vi "demodrive.vi"   [LabVIEW 2012, in "Demo.lvrbt"]
uses:
  Demo.lvrbt
  <vilib>/NXT/Hardware/Plugins/Tetrix DC Motor/TetrixDCMotorAddress.ctl
  <vilib>/FTC/FTC Read Controller Packet.vi
  <vilib>/FTC/FTC Read Button States.vi
  <vilib>/FTC/FTC Calculate Drive Power - Tank.vi
  <vilib>/NXT/NXTIO Xnodes/NXTIONodeSubVIs/TETRIX IO Move DC Motors.vi
  <vilib>/NXT/NXTIO Xnodes/NXTIONodeSubVIs/TETRIX IO Check Battery.vi
  <vilib>/NXT/NXTIO Xnodes/AddressXNode/NXTIOAddress.xnode
  <vilib>/NXT/Subs/LVHSConnector.ctl
  <vilib>/NXT/NXTIO Xnodes/NXTIOXNode/NXTIO.xnode
  <vilib>/NXT/LegoClasses/BrickReference/BrickReference.lvclass
panel:
  # "This VI was generated based on your configuration in the Remote Control Editor. You may modify the code as needed for your robot. To test this program for an FTC match, return to the Remote Control Editor, select the \"Run Program\" tab, and choose \"FTC Game\"."
types:
  T1 = typedef "TetrixDCMotorAddress.ctl" = i16
  T2 = cluster{"TetrixDCMotor":T1, "TetrixDCMotor 2":T1}
  T3 = typedef "LVHSConnector.ctl" = refnum<class "BrickReference.lvclass">
  T4 = typedef "FTC ControllerState.ctl" = cluster{"Left X":i8, "Left Y":i8, "Right X":i8, "Right Y":i8, "Button Encoding 9-12":u8, "Button Encoding 1-8":u8, "POV":T5}
  T5 = typedef "FTC POVState.ctl" = i8
  T6 = typedef "FTC ButtonEventType.ctl" = enum16{"Pressed", "Released"}
  T7 = cluster{"Button ID":enum16{"None", "Button 1", "Button 2", "Button 3", "Button 4", "Button 5", "Button 6", "Button 7", "Button 8", "Button 9", "Button 10", "Button 11", "Button 12", "POV Up", "POV Up Right", "POV Right", "POV Down Right", "POV Down", "POV Down Left", "POV Left", "POV Up Left"}, "Event Type":T6}[]
  T8 = enum16{"None", "Button 1", "Button 2", "Button 3", "Button 4", "Button 5", "Button 6", "Button 7", "Button 8", "Button 9", "Button 10", "Button 11", "Button 12", "POV Up", "POV Up Right", "POV Right", "POV Down Right", "POV Down", "POV Down Left", "POV Left", "POV Up Left"}
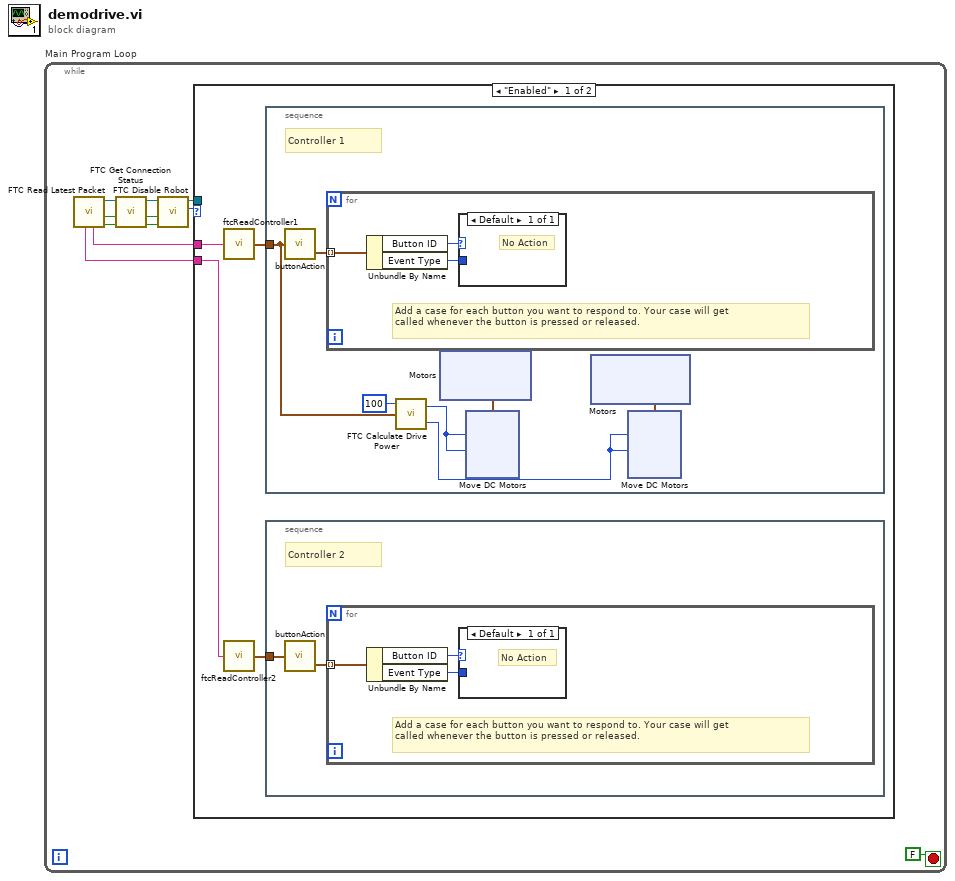
[diagram p0: block diagram]
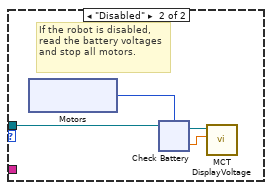
[diagram p2: hidden frame]
diagram:
  n1 = while "Main Program Loop" {
    stop <- FALSE stop-if-true
    n2 = call <vilib>:"FTC Read Latest Packet.vi"() -> ("Packet Received?"=w8:bool, "Stopped?"=w5:bool, "NXT"=w7:T3, "Controller 1"=w10:string, "Controller 2"=w9:string)  [unwired: 6 in, 1 out]
    n3 = call <vilib>:"FTC Get Connection Status.vi"("Packet Received?"=w8, "Stopped?"=w5, "NXT"=w7) -> ("Online?"=w2:bool, "Stopped?"=w3:bool, "NXT"=w4:T3)  [unwired: 5 in]
    n4 = call <vilib>:"FTC Disable Robot.vi"("Online?"=w2, "Stopped?"=w3, "NXT"=w4) -> ("Enabled?"=w6:enum16{"Disabled", "Enabled"}, "NXT"=w1:T3)  [unwired: 3 in]
    n5 = case "disableCase" shown="\"Enabled\"" w6 {
      tunnel: w10 -> [w15 _]
      tunnel: w9 -> [w14 _]
      tunnel: w1 -> [_ w56]
      frame "Enabled" {
        n6 = call "ftcReadController1"("Packet"=w15) -> ("Controller State"=w13:T4)  [unwired: 4 in]
        n7 = call "ftcReadController2"("Packet"=w14) -> ("Controller State"=w12:T4)  [unwired: 4 in]
        n8 = stacked-sequence "controller1Actions" {
          tunnel: w13 -> [w26]
          frame #0 {
            # "Controller 1"
            n9 = call "buttonAction"("Controller State"=w26) -> ("Button Events"=w27:T7)  [unwired: 2 in, 1 out]
            n10 = for "buttonAction" {
              tunnel: w27 -> [w50] mode=indexing
              # "Add a case for each button you want to respond to. Your case will get \ncalled whenever the button is pressed or released."
              n11 = Unbundle By Name(w50) -> ("Button ID"=w52:T8, "Event Type"=w51:T6)
              n12 = case "EventCase1" shown="Default" w52 {
                tunnel: w51 -> [_]
                frame Default {
                  # "No Action"
                }
              }
            }
            n13 = call-poly <vilib>:"FTC Calculate Drive Power.vi"("Controller State"=w26, "Power Level (50)"=i8 100) -> ("Right Motor Power"=w21:i8, "Left Motor Power"=w22:i8)  [unwired: 2 in]
            n14 = xnode "Motors"() -> ("Motor"=w24:cluster{"TetrixDCMotor":T1, "TetrixDCMotor":T1})
            n15 = xnode "Move DC Motors"("Power/Speed 2"=w22, "Power/Speed 1"=w22, "Motors"=w24) -> ()  [unwired: 1 in, 1 out]
            n16 = xnode "Motors"() -> ("Motor"=w23:cluster{"TetrixDCMotor":T1, "TetrixDCMotor":T1})
            n17 = xnode "Move DC Motors"("Power/Speed 2"=w21, "Power/Speed 1"=w21, "Motors"=w23) -> ()  [unwired: 1 in, 1 out]
          }
        }
        n18 = stacked-sequence "controller2Actions" {
          tunnel: w12 -> [w16]
          frame #0 {
            # "Controller 2"
            n19 = call "buttonAction"("Controller State"=w16) -> ("Button Events"=w17:T7)  [unwired: 2 in, 1 out]
            n20 = for "buttonAction" {
              tunnel: w17 -> [w18] mode=indexing
              # "Add a case for each button you want to respond to. Your case will get \ncalled whenever the button is pressed or released."
              n21 = Unbundle By Name(w18) -> ("Button ID"=w20:T8, "Event Type"=w19:T6)
              n22 = case "EventCase2" shown="Default" w20 {
                tunnel: w19 -> [_]
                frame Default {
                  # "No Action"
                }
              }
            }
          }
        }
      }
      frame "Disabled" {
        # "If the robot is disabled, read the battery voltages and stop all motors."
        n23 = xnode ("Motors")() -> ("Motor"=w55:T1)
        n24 = xnode "Check Battery"("Motors"=w55, "NXT"=w56) -> ("Voltage 1"=w54:sgl, "NXT"=w53:T3)
        n25 = call <vilib>:"MCT DisplayVoltage.vi"("Motor Voltage"=w54, "NXT"=w53) -> ()  [unwired: 9 in, 1 out]
      }
    }
  }
